vi "Create GUID.vi"(10 "error in (no error)":errorcluster) -> (2 "error out":errorcluster, 3 "GUID":string)   [LabVIEW 2011, in "COSYLib.lvlib"]
uses:
  COSYLib.lvlib
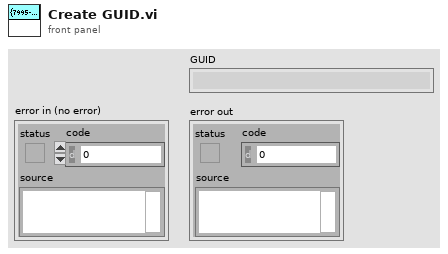
[diagram p1: front panel]
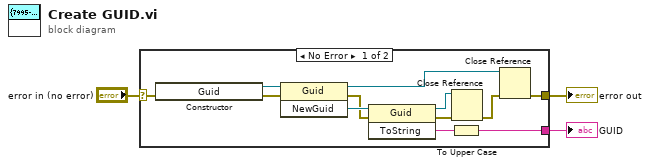
[diagram p0: block diagram]
diagram:
  n1 = case shown="No Error" "error in (no error)" {
    selector: "error in (no error)" -> [w4 w16]
    tunnel: [w7 w16] -> w3
    tunnel: [w5 _] -> w2
    frame No Error {
      n2 = constructor class="System.Guid" ("Constructor Node")(error in=w4) -> (reference out=w15:refnum<k24>, error out=w14:errorcluster)  [unwired: 2 in, 1 out]
      n3 = invoke class="Guid" method="NewGuid"(reference=w15, error in=w14) -> (reference out=w9:refnum<k24>, error out=w12:errorcluster, "NewGuid"=w13:refnum<k24>)  [unwired: 1 in]
      n4 = invoke class="Guid" method="ToString"(reference=w13, error in=w12) -> (reference out=w10:refnum<k24>, error out=w11:errorcluster, "ToString"=w6:string)  [unwired: 1 in]
      n5 = To Upper Case(1:w6) -> (0:w5:string)
      n6 = Close Reference(reference=w10, error in (no error)=w11) -> (error out=w8:errorcluster)
      n7 = Close Reference(reference=w9, error in (no error)=w8) -> (error out=w7:errorcluster)
    }
    frame Error {
    }
  }
  "error out" <- w3
  "GUID" <- w2
